vi "DSF.Shared.Constants.vi"   [LabVIEW 2017, in "Data Sharing Framework Engine.lvlib"]
uses:
  Source/Data Sharing Framework Core/Engine/Data Sharing Framework Engine.lvlib
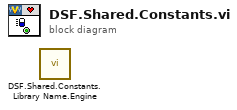
[diagram p0: block diagram]
diagram:
  n1 = call "DSF.Shared.Constants.Library Name.Engine.vi"() -> ()  [unwired: 11 in, 1 out]
